vi "Create File (SubVI).vi"(2 "error in":errorcluster caption="error in (no error)", 3 "headers":string, 4 "data name":string, 5 "file name":string) -> (0 "error out":errorcluster, 1 "Byte Stream File out":refnum<file>)   [LabVIEW 2017]
doc: "by Tanguy BOULARD"
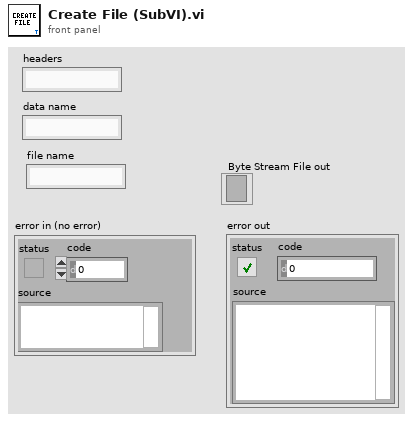
[diagram p1: front panel]
types:
  T1 = enum16{"open", "replace", "create", "open or create", "replace or create", "replace or create with confirmation"}
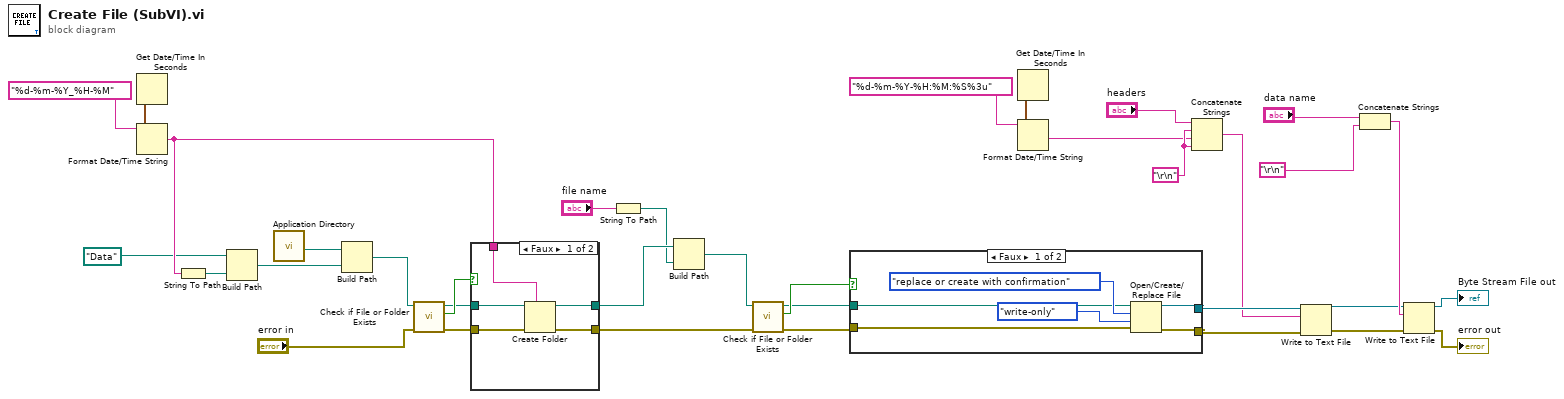
[diagram p0: block diagram]
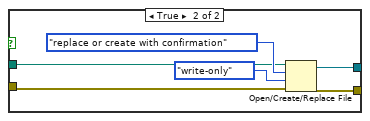
[diagram p3: hidden frame]
diagram:
  w12 = "\r\n"
  n1 = Get Date/Time In Seconds() -> (seconds since 1Jan1904=w30:timestamp)
  n2 = Format Date/Time String(time format string (%c)="%d-%m-%Y_%H-%M", seconds (now)=w30) -> (date/time string=w4:string)  [unwired: 1 in]
  n3 = String To Path(string=w4) -> (path=w3:path)
  n4 = Build Path(base path=path "Data", name or relative path=w3) -> (appended path=w2:path)
  n5 = call <vilib>:"Application Directory.vi"() -> ("Application Directory"=w28:path)
  n6 = Build Path(base path=w28, name or relative path=w2) -> (appended path=w24:path)
  n7 = call <vilib>:"Check if File or Folder Exists.vi"("error in (no error)"="error in", "path"=w24) -> ("error out"=w22:errorcluster, "file or folder exists?"=w23:bool, "dup path"=w21:path)  [unwired: 7 in]
  n8 = case shown="Faux" w23 {
    tunnel: w22 -> [w38 w42]
    tunnel: [w37 w42] -> w15
    tunnel: w21 -> [w40 w41]
    tunnel: [w39 w41] -> w19
    tunnel: w4 -> [w36 _]
    frame False {
      n9 = Create Folder(prompt (Create Folder)=w36, path (use dialog)=w40, error in=w38) -> (created path=w39:path, error out=w37:errorcluster)  [unwired: 1 out]
    }
    frame True {
    }
  }
  n10 = String To Path(string="file name") -> (path=w17:path)
  n11 = Build Path(base path=w19, name or relative path=w17) -> (appended path=w16:path)
  n12 = call <vilib>:"Check if File or Folder Exists.vi"("error in (no error)"=w15, "path"=w16) -> ("error out"=w14:errorcluster, "file or folder exists?"=w20:bool, "dup path"=w13:path)  [unwired: 7 in]
  n13 = case shown="Faux" w20 {
    tunnel: [w45 w49] -> w35
    tunnel: [w46 w50] -> w32
    tunnel: w13 -> [w44 w52]
    tunnel: w14 -> [w43 w51]
    frame False {
      n14 = Open/Create/Replace File(file path (use dialog)=w44, error in=w43, operation (0:open)=T1."replace or create with confirmation", access (0:read/write)=enum16{"read/write", "read-only", "write-only"}."write-only") -> (refnum out=w45:refnum<file>, error out=w46:errorcluster)  [unwired: 2 in, 1 out]
    }
    frame True {
      n15 = Open/Create/Replace File(file path (use dialog)=w52, error in=w51, operation (0:open)=T1."replace or create with confirmation", access (0:read/write)=enum16{"read/write", "read-only", "write-only"}."write-only") -> (refnum out=w49:refnum<file>, error out=w50:errorcluster)  [unwired: 2 in, 1 out]
    }
  }
  n16 = Get Date/Time In Seconds() -> (seconds since 1Jan1904=w7:timestamp)
  n17 = Format Date/Time String(time format string (%c)="%d-%m-%Y-%H:%M:%S%3u", seconds (now)=w7) -> (date/time string=w5:string)  [unwired: 1 in]
  n18 = Concatenate Strings("headers", w12, w5, w12) -> (w34:string)
  n19 = Write to Text File(file (use dialog)=w35, text=w34, error in=w32) -> (refnum out=w10:refnum<file>, error out=w11:errorcluster)  [unwired: 1 in, 1 out]
  n20 = Concatenate Strings("data name", "\r\n") -> (w27:string)
  n21 = Write to Text File(file (use dialog)=w10, text=w27, error in=w11) -> (refnum out=→"Byte Stream File out":refnum<file>, error out=→"error out":errorcluster)  [unwired: 1 in, 1 out]
